vi "Cheezy Drive control.vi"(10 "Throttle":dbl, 11 "Steer":dbl) -> (2 "Right motor output":dbl, 3 "Left motor ouput":dbl)   [LabVIEW 2013]
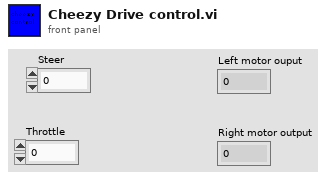
[diagram p1: front panel]
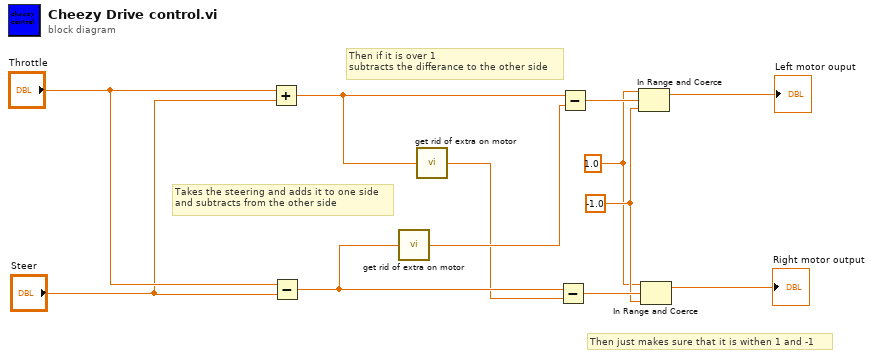
[diagram p0: block diagram]
diagram:
  w3 = -1.0 ("lower limit")
  w2 = 1.0 ("upper limit")
  # "Then just makes sure that it is withen 1 and -1"
  # "Then if it is over 1\nsubtracts the differance to the other side"
  # "Takes the steering and adds it to one side\nand subtracts from the other side"
  n1 = Add(x="Throttle", y="Steer") -> (x+y=w8:dbl)
  n2 = Subtract(x="Throttle", y="Steer") -> (x-y=w10:dbl)
  n3 = call "get rid of extra on motor.vi"("Numeric"=w10) -> ("extra"=w9:dbl)
  n4 = call "get rid of extra on motor.vi"("Numeric"=w8) -> ("extra"=w7:dbl)
  n5 = Subtract(x=w10, y=w7) -> (x-y=w4:dbl)
  n6 = Subtract(x=w8, y=w9) -> (x-y=w6:dbl)
  n7 = In Range and Coerce(upper limit=w2, x=w6, lower limit=w3) -> (coerced(x)=→"Left motor ouput":dbl)  [unwired: 1 out]
  n8 = In Range and Coerce(upper limit=w2, x=w4, lower limit=w3) -> (coerced(x)=→"Right motor output":dbl)  [unwired: 1 out]
